vi "Authentication.vi"(8 "error in (no error)":errorcluster, 11 "Hello in":refnum<class "Hello.lvclass">) -> (0 "error out":errorcluster, 2 "Authentication":T1, 3 "Hello out":refnum<class "Hello.lvclass">)   [LabVIEW 2020, in "obs-websocket.lvlib" / "Hello.lvclass"]
uses:
  Hello.lvclass
  Authentication.ctl
  Hello.lvclass/Hello.ctl
  obs-websocket.lvlib
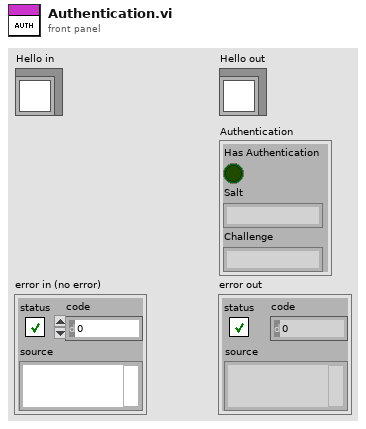
[diagram p1: front panel]
types:
  T1 = typedef "obs-websocket.lvlib/Authentication.ctl" = cluster{"Has Authentication":bool, "Salt":string, "Challenge":string}
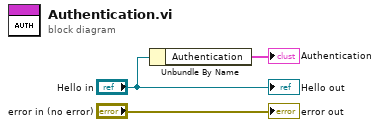
[diagram p0: block diagram]
diagram:
  n1 = Unbundle By Name("Hello in") -> ("Authentication"=→"Authentication":T1)
  "error out" <- "error in (no error)"
  "Hello out" <- "Hello in"
